vi "parse_channel_float32.vi"(4 "error in":errorcluster, 7 "msg in":string) -> (0 "error out":errorcluster, 2 "ChannelFloat32":cluster{"Name":string, "Values":sgl[]}, 3 "msg out":string)   [LabVIEW 2010]
uses:
  primitives/subs/parse_string_scalar.vi
  primitives/subs/parse_float32_array.vi
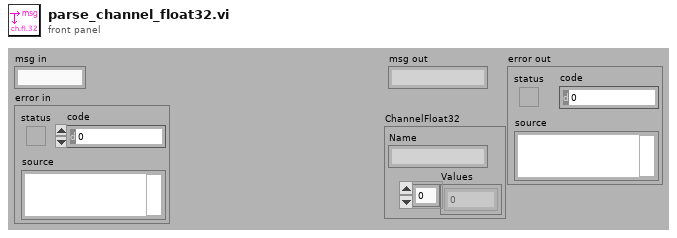
[diagram p1: front panel]
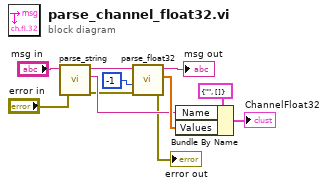
[diagram p0: block diagram]
diagram:
  n1 = call-poly "parse_string.vi"("error in"="error in", "msg in"="msg in") -> ("error out"=w3:errorcluster, "string"=w6:string, "msg out"=w9:string)  [unwired: 3 in]
  n2 = call-poly "parse_float32.vi"("error in"=w3, "Array Size"=-1, "msg in"=w9) -> ("error out"=→"error out":errorcluster, "number"=w8:sgl[], "msg out"=→"msg out":string)  [unwired: 2 in]
  n3 = Bundle By Name(cluster=cluster{"Name":string, "Values":sgl[]} {"Name"="", "Values"=[]} ("Channel 2"), "Name"=w6, "Values"=w8) -> (→"ChannelFloat32":cluster{"Name":string, "Values":sgl[]})
